vi "Extract IRF (Topless).vi"(4 "balance parameter (-1: auto)":dbl=-1.0, 6 "Tail Smoothing (T)":bool=TRUE, 7 "Smoothing Order":i32=1, 8 "Error In":errorcluster, 9 "Time Constant":dbl, 10 "Intensity Array":dbl[](array[numeric]), 11 "t Array":dbl[](array[numeric])) -> (0 "Error Out":errorcluster, 1 "Message":string, 2 "IRF Array":dbl[](array[numeric]), 3 "t Array (dup)":dbl[](array[numeric]))   [LabVIEW 2021, in "Fits.lvlib"]
doc: "Extract IRF from provided decay and time constant"
uses:
  Fits.lvlib
  <vilib>/Analysis/baseanly.llb/Matrix Type of Inverse Matrix.ctl
  <vilib>/Analysis/baseanly.llb/A x Vector.vi
  <vilib>/Analysis/7linalg.llb/Create Special Real Matrix.vi
  <vilib>/Analysis/baseanly.llb/Real Inverse Matrix.vi
  <vilib>/Utility/error.llb/Error Cluster From Error Code.vi
  <vilib>/ErrorRing/Error Ring.xnode
  <vilib>/Analysis/NI_AALPro.lvlib
  <vilib>/Analysis/NI_AALBase.lvlib
  Graphs/XY Graph/XY Graph Add-Ons.lvlib
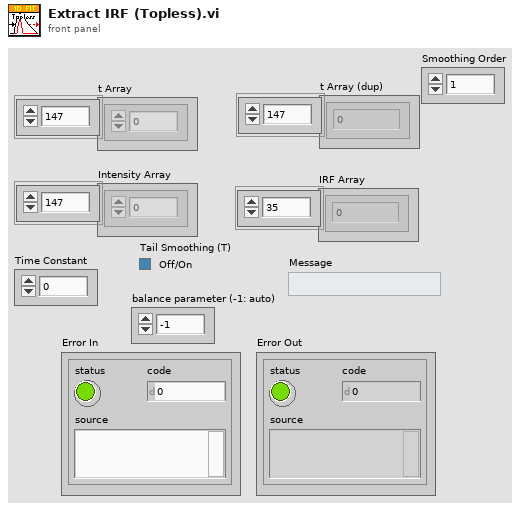
[diagram p1: front panel]
types:
  T1 = typedef "NI_AALBase.lvlib/Matrix Type of Inverse Matrix.ctl" = enum32{"General", "Positive Definite", "Lower Triangular", "Upper Triangular"}
  T2 = typedef "NI_Matrix.lvlib/RealMatrix.ctl" = dbl[][]
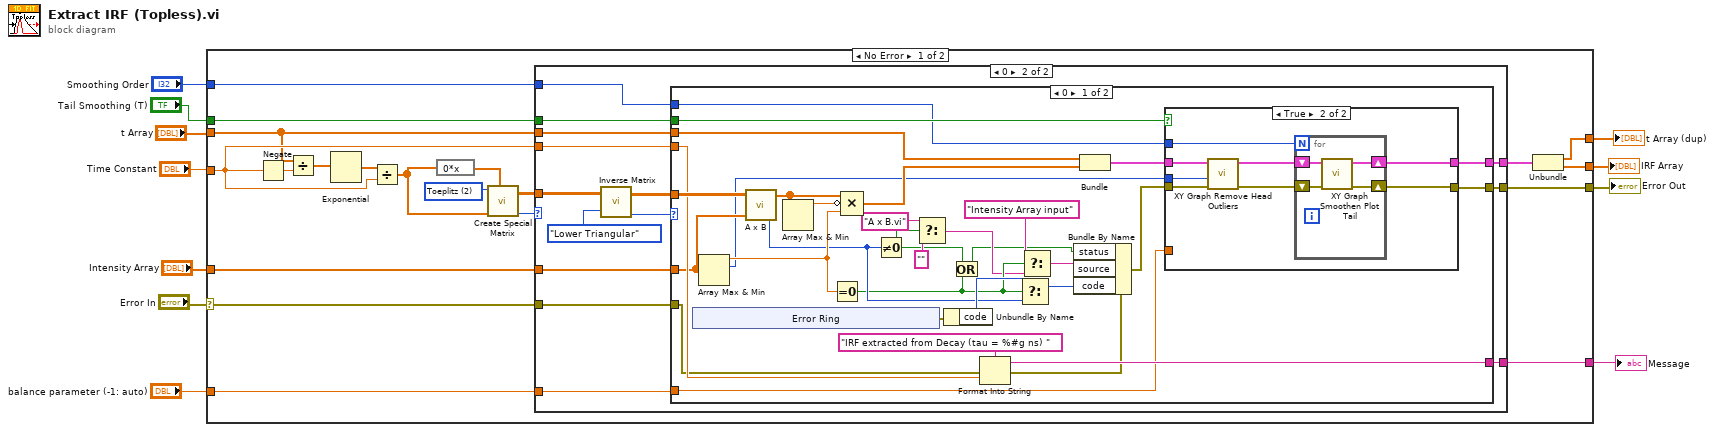
[diagram p0: block diagram]
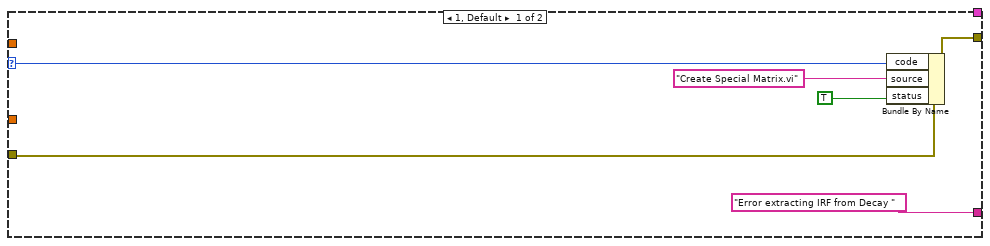
[diagram p2: hidden frame]
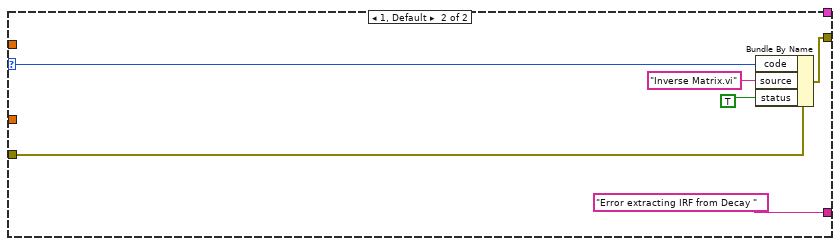
[diagram p4: hidden frame]
diagram:
  n1 = case shown="No Error" "Error In" {
    selector: "Error In" -> [w17 w108]
    tunnel: "Intensity Array" -> [w31 _]
    tunnel: "Time Constant" -> [w21 _]
    tunnel: "t Array" -> [w19 _]
    tunnel: [w16 w108] -> w8
    tunnel: [w22 _] -> w6
    tunnel: "Tail Smoothing (T)" -> [w20 _]
    tunnel: "balance parameter (-1: auto)" -> [w18 _]
    tunnel: [w14 _] -> w3
    tunnel: [w13 _] -> w2
    tunnel: "Smoothing Order" -> [w12 _]
    frame No Error {
      w29 = 2 items=["Identity", "Diagonal", "Toeplitz", "Vandermonde", "Companion", "Hankel", "Hadamard", "Wilkinson", "Hilbert", "Inverse Hilbert", "Rosser", "Pascal"] ("matrix type")
      n2 = Negate(x=w21) -> (-x=w26:dbl)
      n3 = Divide(x=w19, y=w26) -> (x/y=w24:dbl[])
      n4 = Exponential(1:w24) -> (0:w25:dbl[])
      n5 = Divide(x=w25, y=w21) -> (x/y=w28:dbl[])
      n6 = expression code="0*x"(w28) -> (w27:dbl[])
      n7 = call-poly <vilib>:"Create Special Matrix.vi"("matrix type"=w29, "Input Vector1"=w28, "Input Vector2"=w27) -> ("Special Matrix"=w30:T2, "error"=w23:i32)  [unwired: 2 in]
      n8 = case shown="0" w23 {
        selector: w23 -> [w36 _]
        tunnel: w31 -> [_ w51]
        tunnel: w30 -> [_ w49]
        tunnel: ["Error extracting IRF from Decay " ("Message") w46] -> w22
        tunnel: w21 -> [_ w45]
        tunnel: w20 -> [_ w44]
        tunnel: w19 -> [_ w43]
        tunnel: w18 -> [_ w42]
        tunnel: w17 -> [w34 w41]
        tunnel: [w32 w40] -> w16
        tunnel: [_ w39] -> w15
        tunnel: w12 -> [_ w38]
        frame 1, Default {
          n9 = Bundle By Name(cluster=w34, "code"=w36, "source"="Create Special Matrix.vi", "status"=TRUE) -> (w32:errorcluster)
        }
        frame 0 {
          n10 = call-poly <vilib>:"Inverse Matrix.vi"("matrix type"=Matrix_Type_of_Inverse_Matrix."Lower Triangular", "Input Matrix"=w49) -> ("error"=w47:i32, "Inverse Matrix"=w50:T2)
          n11 = case shown="0" w47 {
            selector: w47 -> [_ w106]
            tunnel: w51 -> [w65 _]
            tunnel: w50 -> [w83 _]
            tunnel: [w70 "Error extracting IRF from Decay " ("Message")] -> w46
            tunnel: w45 -> [w68 _]
            tunnel: w44 -> [w67 _]
            tunnel: w43 -> [w64 _]
            tunnel: w42 -> [w62 _]
            tunnel: w41 -> [w53 w103]
            tunnel: [w57 w102] -> w40
            tunnel: [w56 _] -> w39
            tunnel: w38 -> [w55 _]
            frame 0 {
              n12 = xnode "Error Ring"() -> ("error out"=w77:errorcluster)
              n13 = Array Max & Min(array=w65) -> (max value=w78:dbl, max index (indices)=w52:i32)  [unwired: 2 out]
              n14 = call-poly <vilib>:"A x B.vi"("Vector"=w65, "A"=w83) -> ("error"=w75:i32, "A x Vector"=w80:dbl[])
              n15 = Array Max & Min(array=w80) -> (max value=w79:dbl)  [unwired: 3 out]
              n16 = Equal To 0?(x=w78) -> (x = 0?=w74:bool)
              n17 = Compound Arithmetic op=MULTIPLY(w80, invert w79, w78) -> (w66:dbl[])
              n18 = Not Equal To 0?(x=w75) -> (x != 0?=w71:bool)
              n19 = Select(t="A x B.vi", s=w71, f="") -> (s? t:f=w73:string)
              n20 = Unbundle By Name(w77) -> ("code"=w76:i32)
              n21 = Or(x=w71, y=w74) -> (x .or. y?=w59:bool)
              n22 = Format Into String(format string="IRF extracted from Decay (tau = %#g ns) " ("Message"), error in=w53, w68) -> (resulting string=w70:string, error out=w54:errorcluster)  [unwired: 1 in]
              n23 = Select(t=w76, s=w74, f=w75) -> (s? t:f=w60:i32)
              n24 = Select(t="Intensity Array input", s=w74, f=w73) -> (s? t:f=w61:string)
              n25 = Bundle By Name(cluster=w54, "status"=w59, "source"=w61, "code"=w60) -> (w58:errorcluster)
              n26 = Bundle("t Array"=w64, w66) -> (w63:cluster{"t Array":dbl[], dbl[]})  [unwired: 1 in]
              n27 = case shown="True" w67 {
                tunnel: w52 -> [_ w88]
                tunnel: w63 -> [w85 w93]
                tunnel: w62 -> [_ _]
                tunnel: [w85 w92] -> w56
                tunnel: w58 -> [w84 w86]
                tunnel: [w84 w91] -> w57
                tunnel: w55 -> [_ w90]
                frame False {
                }
                frame True {
                  n28 = call "XY Graph Remove Head Outliers.vi"("Error In"=w86, "Peak Index (-1: unknown)"=w88, "Plot in"=w93) -> ("Error Out"=w87:errorcluster, "Plot out"=w89:cluster{"t Array":dbl[], "Array":dbl[]})  [unwired: 6 in, 1 out]
                  n29 = for {
                    N: w90 -> [_]
                    shift-right: [w95] -> w92
                    shift-left: w89 -> [w97]
                    shift-right: [w94] -> w91
                    shift-left: w87 -> [w96]
                    n30 = call "XY Graph Smoothen Plot Tail.vi"("error in (no error)"=w96, "Plot in"=w97) -> ("error out"=w94:errorcluster, "Plot out"=w95:cluster{"t Array":dbl[], "Y Array":dbl[]})  [unwired: 8 in]
                  }
                }
              }
            }
            frame 1, Default {
              n31 = Bundle By Name(cluster=w103, "code"=w106, "source"="Inverse Matrix.vi", "status"=TRUE) -> (w102:errorcluster)
            }
          }
        }
      }
      n32 = Unbundle(w15) -> ("t Array"=w14:dbl[], "Array"=w13:dbl[])
    }
    frame Error {
    }
  }
  "IRF Array" <- w2
  "Error Out" <- w8
  "t Array (dup)" <- w3
  "Message" <- w6
